vi "Languages.vi"(10 "Pict Ring":u16(ring)) -> ()   [LabVIEW 2020]
panel:
  in  "Pozisyon (Position)":dbl caption="Pozisyon" format="%#_g mm"
  in  "Kuvvet (Force)":dbl caption="Kuvvet" format="%#_6g N"
  in  "bt_testCall":bool caption="Test Çağır"
  in  "bt_stopHydraulicSystem":bool caption="Sistem Durdur"
  in  "bt_startHydraulicSystem":bool caption="Sistem Başlat"
  out "Display Message":string="Test Edit" caption="DURUM BİLGİSİ"
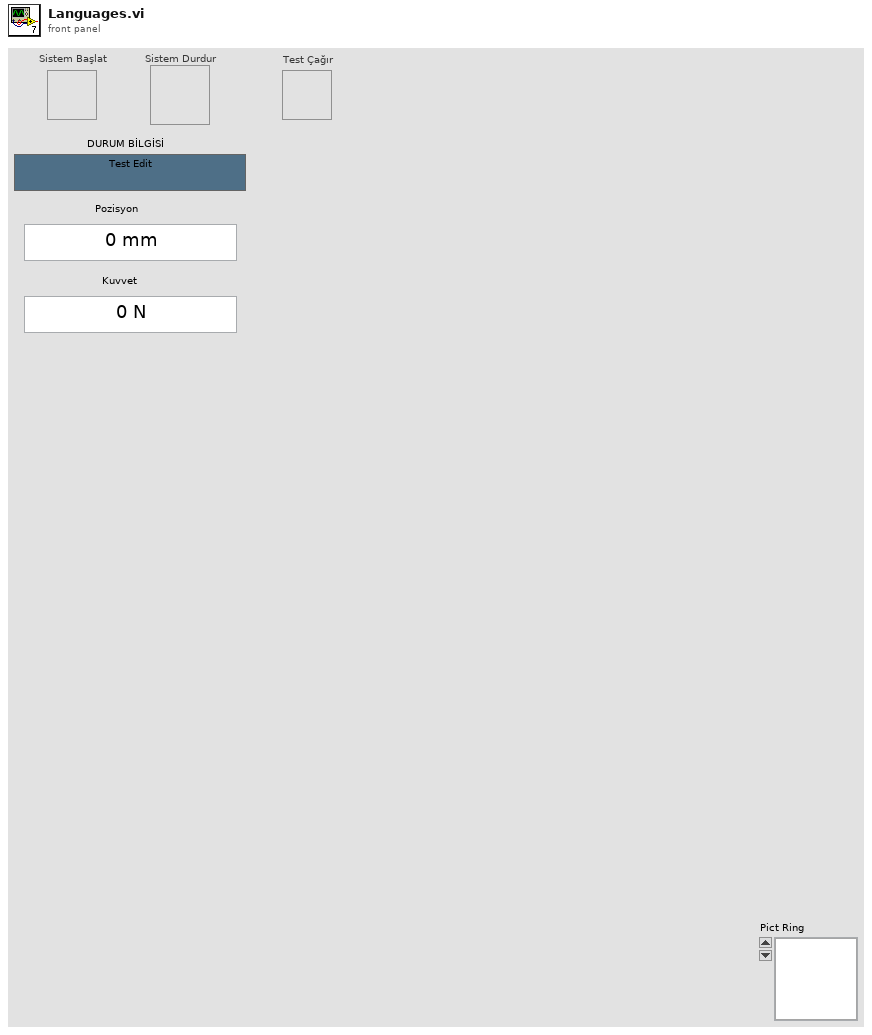
[diagram p1: front panel]
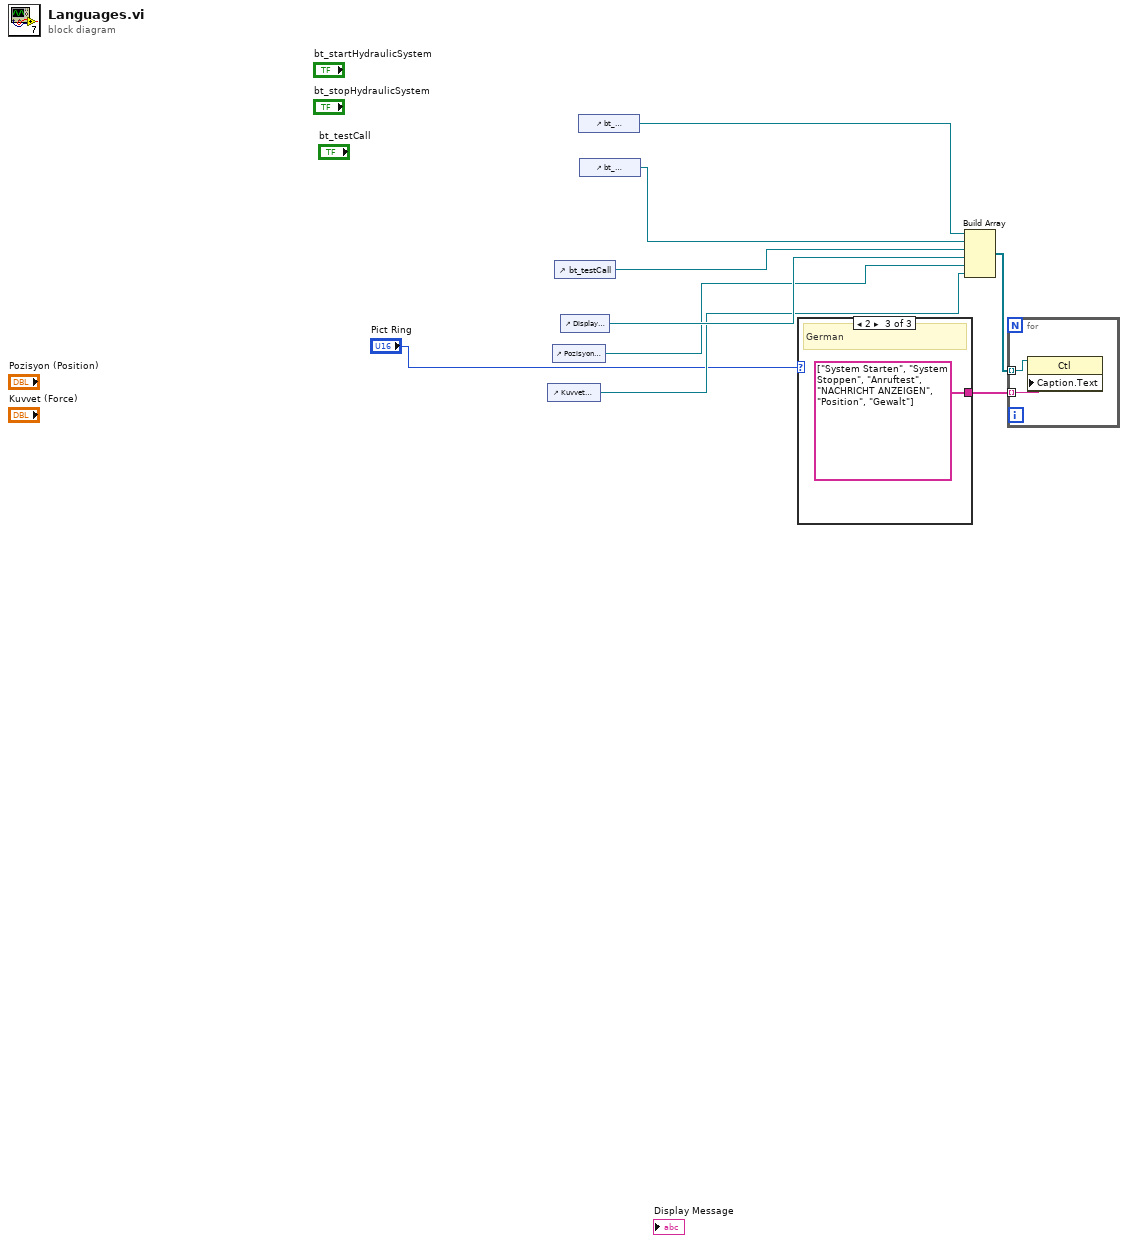
[diagram p0: block diagram]
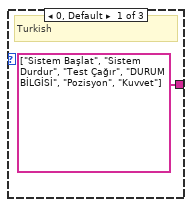
[diagram p2: hidden frame]
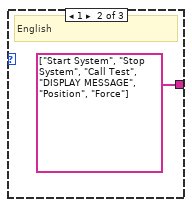
[diagram p3: hidden frame]
diagram:
  n1 = control-ref of="Kuvvet (Force)"() -> (w2:refnum<vi>)
  n2 = control-ref of="Pozisyon (Position)"() -> (w3:refnum<vi>)
  n3 = control-ref of="bt_testCall"() -> (w5:refnum<vi>)
  n4 = control-ref of="Display Message"() -> (w4:refnum<vi>)
  n5 = control-ref of="bt_startHydraulicSystem"() -> (w7:refnum<vi>)
  n6 = control-ref of="bt_stopHydraulicSystem"() -> (w6:refnum<vi>)
  n7 = case shown="2" "Pict Ring" {
    tunnel: [string[] ["Sistem Başlat", "Sistem Durdur", "Test Çağır", "DURUM BİLGİSİ", "Pozisyon", "Kuvvet"] ("appended array") string[] ["Start System", "Stop System", "Call Test", "DISPLAY MESSAGE", "Position", "Force"] ("appended array") string[] ["System Starten", "System Stoppen", "Anruftest", "NACHRICHT ANZEIGEN", "Position", "Gewalt"] ("appended array")] -> w8
    frame 0, Default {
      # "Turkish"
    }
    frame 1 {
      # "English"
    }
    frame 2 {
      # "German"
    }
  }
  n8 = Build Array(w7, w6, w5, w4, w3, w2) -> (w9:refnum<vi>[])
  n9 = for {
    tunnel: w9 -> [w13] mode=indexing
    tunnel: w8 -> [w14] mode=indexing
    n10 = property class="Ctl"(reference=w13, "Caption.Text"=w14) -> ()  [unwired: 1 in, 2 out]
  }
